vi "test_Basic Waveform Read.vi"(8 "error in (no error)":errorcluster, 11 "DMA Channels Basic Testing in":refnum<class "DMA Channels Basic Testing.lvclass">) -> (0 "error out":errorcluster, 3 "DMA Channels Basic Testing out":refnum<class "DMA Channels Basic Testing.lvclass">)   [LabVIEW 2019, in "DMA Channels Basic Testing.lvclass"]
uses:
  DMA Channels Basic Testing.lvclass
panel:
  out "Waveform":waveform(dbl)(graph)
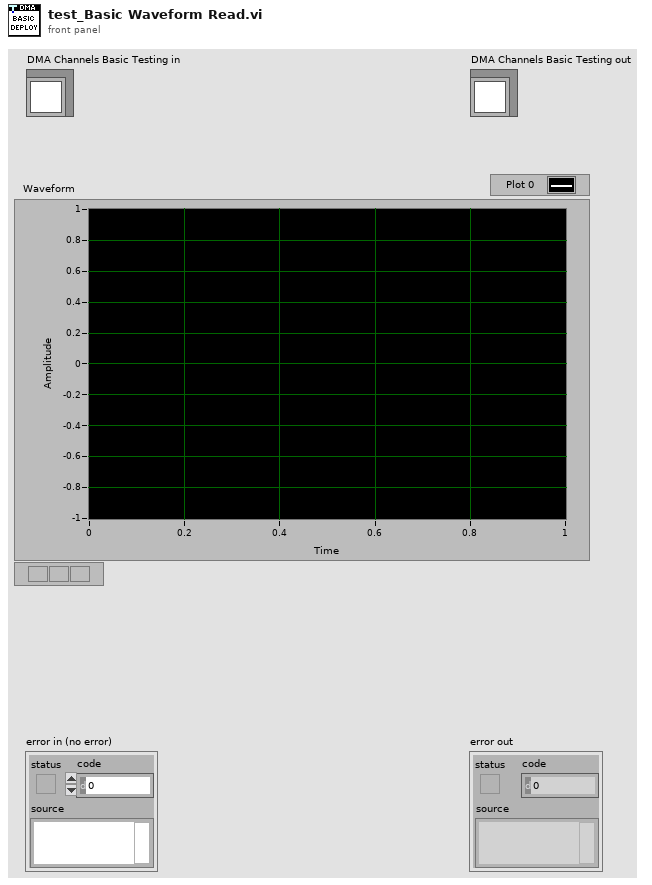
[diagram p1: front panel]
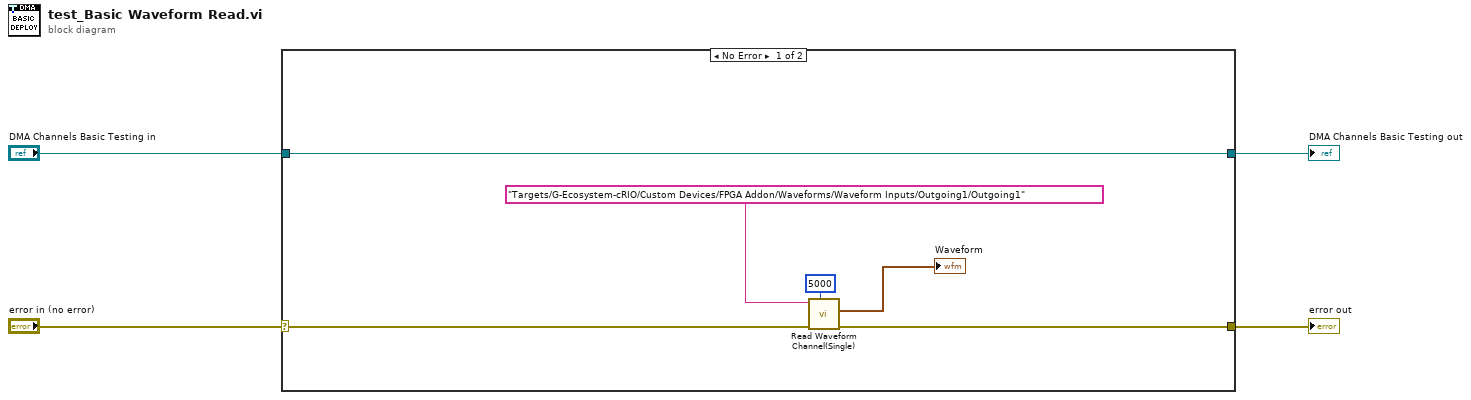
[diagram p0: block diagram]
diagram:
  n1 = case shown="No Error" "error in (no error)" {
    selector: "error in (no error)" -> [w5 w11]
    tunnel: "DMA Channels Basic Testing in" -> [w7 w12]
    tunnel: [w7 w12] -> w3
    tunnel: [w6 w11] -> w2
    frame No Error {
      n2 = call "Read Waveform Channel(Single).vi"("Timeout"=5000, "error in (no error)"=w5, "Waveform path in"="Targets/G-Ecosystem-cRIO/Custom Devices/FPGA Addon/Waveforms/Waveform Inputs/Outgoing1/Outgoing1" ("waveform path")) -> ("error out"=w6:errorcluster, "Waveform data"=→"Waveform":waveform(dbl))  [unwired: 6 in, 1 out]
    }
    frame Error {
    }
  }
  "error out" <- w2
  "DMA Channels Basic Testing out" <- w3
